vi "NewPower_Init.vi"(2 "error in":errorcluster, 3 "Language":T1, 4 "power485":refnum<visa-resource-name>="COM3") -> (0 "error out":errorcluster, 1 "Message":string)   [LabVIEW 2015]
uses:
  CustomControl/Lang_Control.ctl
  <vilib>/Instr/_visa.llb/VISA Configure Serial Port (Instr).vi
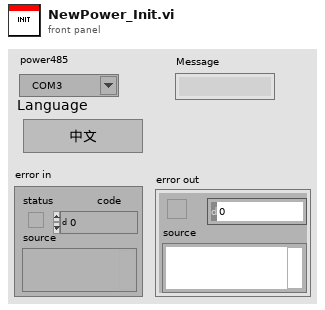
[diagram p1: front panel]
types:
  T1 = typedef "Lang_Control.ctl" = enum16{"中文", "English"}
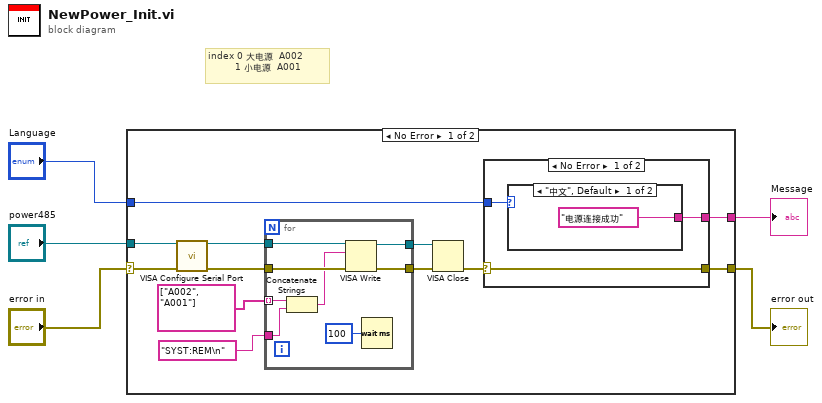
[diagram p0: block diagram]
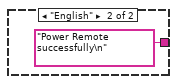
[diagram p2: hidden frame]
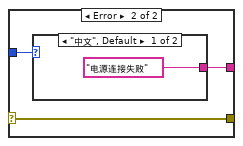
[diagram p3: hidden frame]
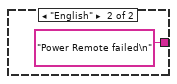
[diagram p4: hidden frame]
diagram:
  # "index 0 大电源  A002\n         1 小电源  A001"
  n1 = case shown="No Error" "error in" {
    selector: "error in" -> [w10 w36]
    tunnel: "power485" -> [w17 _]
    tunnel: [w8 w36] -> w4
    tunnel: [w7 _] -> w2
    tunnel: "Language" -> [w6 _]
    frame No Error {
      n2 = call-poly "VISA Configure Serial Port"("VISA resource name"=w17, "error in (no error)"=w10) -> ("VISA resource name out"=w16:refnum<visa-resource-name>, "error out"=w15:errorcluster)  [unwired: 12 in]
      n3 = for {
        tunnel: w16 -> [w35]
        tunnel: w15 -> [w34]
        tunnel: string[] ["A002", "A001"] -> [w33] mode=indexing
        tunnel: "SYST:REM\n" -> [w32]
        tunnel: [w30] -> w12
        tunnel: [w29] -> w13
        n4 = Concatenate Strings(w33, w32) -> (w31:string)
        n5 = VISA Write(VISA resource name=w35, write buffer=w31, error in (no error)=w34) -> (VISA resource name out=w30:refnum<visa-resource-name>, error out=w29:errorcluster)  [unwired: 1 out]
        n6 = Wait (ms)(milliseconds to wait=u32 100) -> ()  [unwired: 1 out]
      }
      n7 = VISA Close(VISA resource name=w12, error in (no error)=w13) -> (error out=w9:errorcluster)
      n8 = case shown="No Error" w9 {
        selector: w9 -> [w20 w25]
        tunnel: [w20 w25] -> w8
        tunnel: [w19 w24] -> w7
        tunnel: w6 -> [w18 w23]
        frame No Error {
          n9 = case shown="\"中文\", Default" w18 {
            tunnel: ["电源连接成功" "Power Remote successfully\n"] -> w19
            frame "中文", Default {
            }
            frame "English" {
            }
          }
        }
        frame Error {
          n10 = case shown="\"中文\", Default" w23 {
            tunnel: ["电源连接失败" "Power Remote failed\n"] -> w24
            frame "中文", Default {
            }
            frame "English" {
            }
          }
        }
      }
    }
    frame Error {
    }
  }
  "error out" <- w4
  "Message" <- w2
